vi "Text to enum Ring.vi"() -> ()   [LabVIEW 2019]
uses:
  <vilib>/Utility/file.llb/Read Delimited Spreadsheet (string).vi
panel:
  in  "file path (dialog if empty)":path=path "F:/TFS-Labview/My NI 2019/TCSS_V1.0-2023.08.27-Test/TCSS/TCSS/TCSS/TCSS Project/TCSS/Sub VI/ILS/Alarm.csv"
  out "Address":string[][](array[string])
  out "appended array":string[](array[string])
  in  "Public cmd":u16(ring)
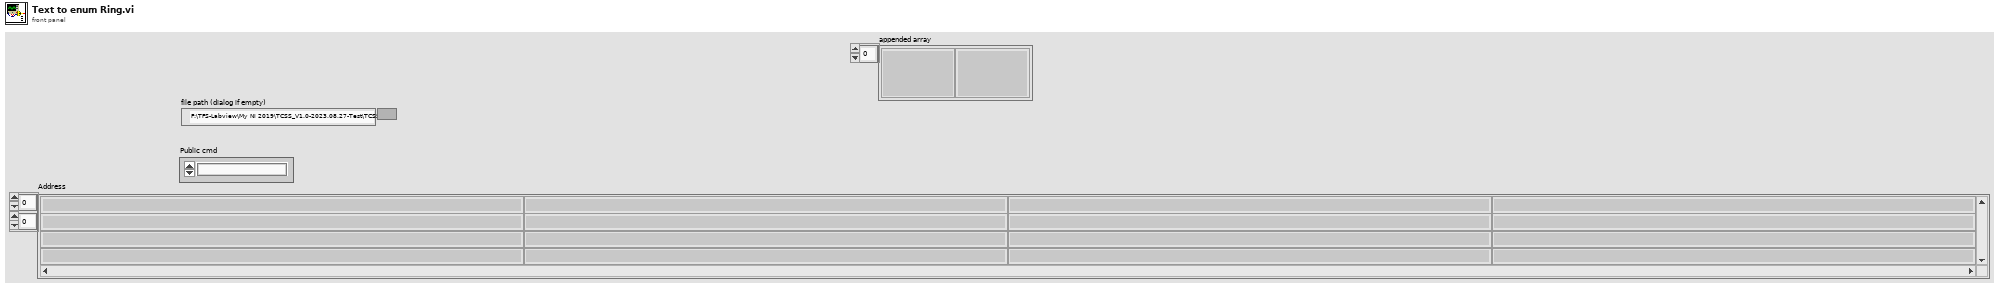
[diagram p1: front panel]
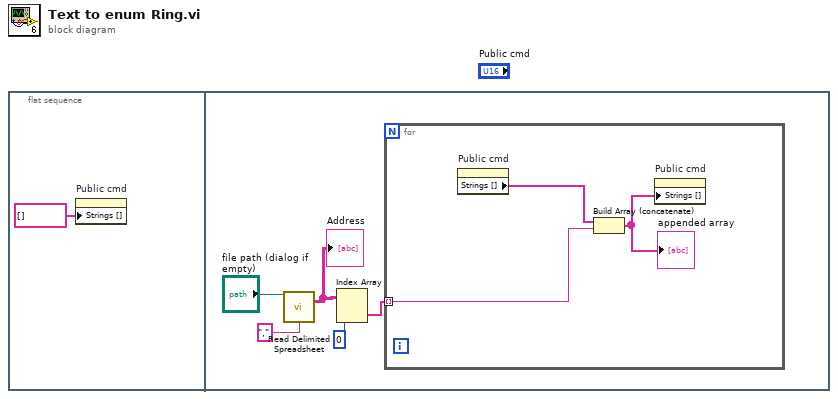
[diagram p0: block diagram]
diagram:
  n1 = flat-sequence {
    frame #0 {
      n2 = property on="Public cmd" class="Ring (strict)"("Strings []"=string[] []) -> ()  [unwired: 2 in, 2 out]
    }
    frame #1 {
      n3 = call-poly <vilib>:"Read Delimited Spreadsheet.vi"("file path (dialog if empty)"="file path (dialog if empty)", "delimiter (\\t)"="," ("delimiter (\\t)")) -> ("all rows"=w3:string[][])  [unwired: 8 in, 5 out]
      "Address" <- w3
      n4 = Index Array(array=w3, index (col)=0 ("disabled index (col)")) -> (element=w4:string[])  [unwired: 1 in]
      n5 = for {
        tunnel: w4 -> [w7] mode=indexing
        n6 = property on="Public cmd" class="Ring (strict)"() -> ("Strings []"=w8:string[])  [unwired: 2 in, 2 out]
        n7 = Build Array (concatenate)(w8, w7) -> (w9:string[])
        "appended array" <- w9
        n8 = property on="Public cmd" class="Ring (strict)"("Strings []"=w9) -> ()  [unwired: 2 in, 2 out]
      }
    }
  }
